vi "ExposeGetRefnumVariantValueOrNull.vi"(9 "Get default value ? (f)":bool, 11 "Data Value Reference in":refnum<data-value>) -> (0 "IsControl":bool, 1 "Control":refnum<vi>, 3 "Data Value Reference Out":refnum<data-value>)   [LabVIEW 2017]
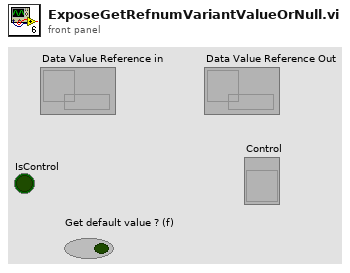
[diagram p1: front panel]
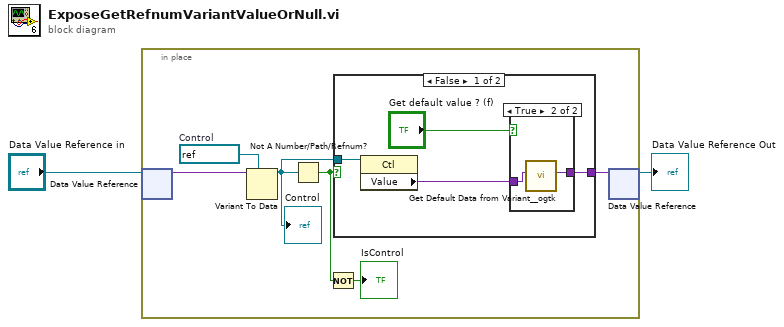
[diagram p0: block diagram]
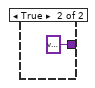
[diagram p3: hidden frame]
diagram:
  n1 = in-place {
    w6 = refnum<vi> refnum  # Control
    n2 = in-place-dvr #1("Data Value Reference in") -> (w4:variant)  [unwired: 1 out]
    n3 = Variant To Data(type=w6, Variant=w4) -> (data=w8:refnum<vi>)  [unwired: 1 in, 1 out]
    "Control" <- w8
    n4 = Not A Number/Path/Refnum?(number/path/refnum=w8) -> (NaN/Path/Refnum?=w7:bool)
    n5 = Not(x=w7) -> (.not. x?=→"IsControl":bool)
    n6 = case shown="False" w7 {
      tunnel: w8 -> [w12 _]
      tunnel: [w10 variant ("Value")] -> w3
      frame False {
        n7 = property class="Ctl"(reference=w12) -> ("Value"=w11:variant)  [unwired: 1 in, 2 out]
        n8 = case shown="True" "Get default value ? (f)" {
          tunnel: w11 -> [w13 w15]
          tunnel: [w13 w14] -> w10
          frame False {
          }
          frame True {
            n9 = call <userlib>:"Get Default Data from Variant__ogtk.vi"("Variant"=w15) -> ("Default VData"=w14:variant)  [unwired: 9 in, 1 out]
          }
        }
      }
      frame True {
      }
    }
    n10 = in-place-dvr #1(w3) -> (→"Data Value Reference Out":refnum<data-value>)  [unwired: 1 out]
  }
